vi "OpenAllNodes.vi"() -> (2 "Nodes":string[][](array[string]))   [LabVIEW 2010]
uses:
  <userlib>/ROSforLV_0.1/ROS/Code/SubVIs/_ROSControl.ctl
  <userlib>/ROSforLV_0.1/ROS/Code/SubVIs/_ROSDirection.ctl
  <userlib>/ROSforLV_0.1/ROS/Code/_ROSDefinition.vi
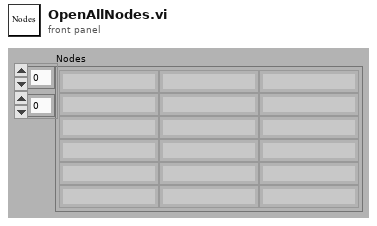
[diagram p1: front panel]
types:
  T1 = typedef "_ROSControl.ctl" = cluster{"topic port":u16, "Node":string, "topic":string, "type":string, "node port":u32, "error ":errorcluster, "Direction":T2, "APIs":string[]}
  T2 = typedef "_ROSDirection.ctl" = enum16{"Node", "Publisher", "Subscriber", "Service Client"}
  T3 = cluster{"server vi":string, "reference":refnum<vi>, "Description":string[]}[]
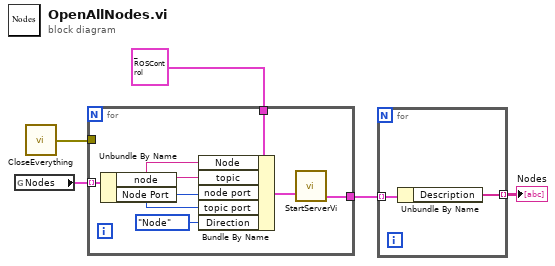
[diagram p0: block diagram]
diagram:
  n1 = global read "_ROSDefinition.vi" "Nodes"() -> (w5:cluster{"node":string, "Node Port":u32}[])
  n2 = call <userlib>:"CloseEverything.vi"() -> ("error out"=w3:errorcluster)  [unwired: 1 in]
  n3 = for {
    tunnel: w5 -> [w12] mode=indexing
    tunnel: T1 {"topic port"=0, "Node"="", "topic"="", "type"="", "node port"=0, "error "={"status"=FALSE, "code"=0, "source"=""}, "Direction"=enum."Node", "APIs"=[]} ("Baxter") -> [w10]
    tunnel: w3 -> [_]
    tunnel: [w6] -> w2
    n4 = Unbundle By Name(w12) -> ("node"=w8:string, "Node Port"=w7:u32)
    n5 = Bundle By Name(cluster=w10, "Node"=w8, "topic"=w8, "node port"=w7, "topic port"=w7, "Direction"=_ROSDirection."Node") -> (w11:T1)
    n6 = call <userlib>:"StartServerVi.vi"("Baxter"=w11) -> ("Active Topics"=w6:T3)  [unwired: 2 out]
  }
  n7 = for {
    tunnel: w2 -> [w14] mode=indexing
    tunnel: [w13] -> w1 mode=indexing
    n8 = Unbundle By Name(w14) -> ("Description"=w13:string[])
  }
  "Nodes" <- w1
